vi "Framework_Initialize.vi"(8 "error in (no error)":errorcluster, 11 "AB_Deploy_EXE in":refnum<class "AB_Deploy_EXE.lvclass">) -> (0 "error out":errorcluster, 1 "helpTopics":string[](array[string]), 2 "pageTitles":string[](array[string]), 3 "AB_Deploy_EXE out":refnum<class "AB_Deploy_EXE.lvclass">, 4 "helpFile":string, 5 "pages":path[](array[path]))   [LabVIEW 2020, in "AB_Deploy_EXE.lvclass"]
uses:
  <vilib>/AppBuilder/AB_Classes/DeployableEXE/AB_Deploy_EXE.lvclass
  <vilib>/AppBuilder/AB_Classes/DeployableEXE/AB_Deploy_EXE.lvclass/AB_Deploy_EXE.ctl
  <vilib>/AppBuilder/AB_Classes/EXE/AB_EXE.lvclass
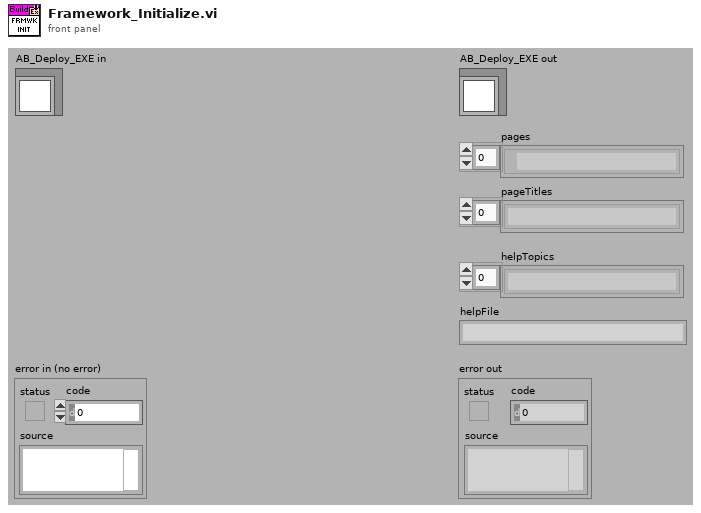
[diagram p1: front panel]
types:
  T1 = enum32{"invalid OS target", "Mac OS", "Windows 3.1", "Windows 95/NT", "Solaris 1", "Solaris 2", "HP-UX", "PowerMAX", "Linux", "Irix", "Rhapsody", "BeOS", "AIX", "OSF1", "VxWorks", "PharLap", "Carbon", "RTX", "Windows x64", "Linux x64", "Mac OS X x64"}
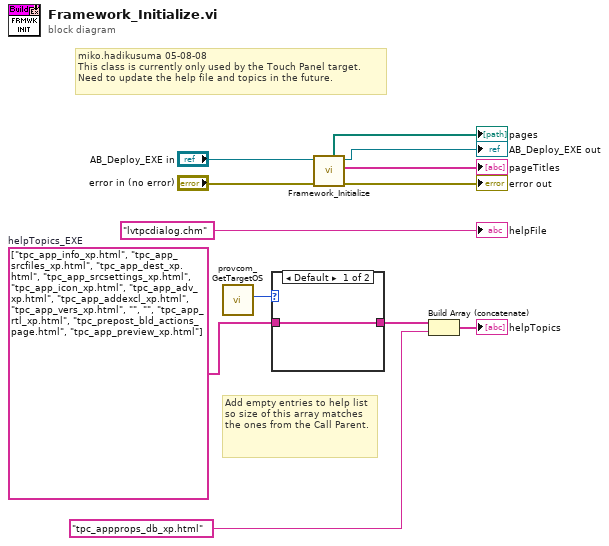
[diagram p0: block diagram]
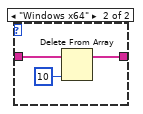
[diagram p2: hidden frame]
diagram:
  w2 = string[] ["tpc_app_info_xp.html", "tpc_app_srcfiles_xp.html", "tpc_app_dest_xp.html", "tpc_app_srcsettings_xp.html", "tpc_app_icon_xp.html", "tpc_app_adv_xp.html", "tpc_app_addexcl_xp.html", "tpc_app_vers_xp.html", "", "", "tpc_app_rtl_xp.html", "tpc_prepost_bld_actions_page.html", "tpc_app_preview_xp.html"]  # helpTopics_EXE
  # "Add empty entries to help list so size of this array matches the ones from the Call Parent."
  # "miko.hadikusuma 05-08-08\nThis class is currently only used by the Touch Panel target.\nNeed to update the help file and topics in the future."
  n1 = call <resource>:"provcom_GetTargetOS.vi"() -> ("App.TargetOS"=w3:T1)  [unwired: 11 out]
  n2 = case shown="Default" w3 {
    tunnel: w2 -> [w13 w16]
    tunnel: [w13 w15] -> w1
    frame Default {
    }
    frame "Windows x64" {
      n3 = Delete From Array(array=w16, index=10) -> (array with subset deleted=w15:string[])  [unwired: 1 in, 1 out]
    }
  }
  n4 = call-parent "Framework_Initialize.vi"("error in (no error)"="error in (no error)", "AB_EXE in"="AB_Deploy_EXE in") -> ("error out"=→"error out":errorcluster, "pageTitles"=→"pageTitles":string[], "AB_EXE out"=→"AB_Deploy_EXE out":refnum<class "AB_Deploy_EXE.lvclass">, "pages"=→"pages":path[])  [unwired: 6 out]
  n5 = Build Array (concatenate)(w1, "tpc_appprops_db_xp.html" ("HTML filename")) -> (→"helpTopics":string[])
  "helpFile" <- "lvtpcdialog.chm" ("CHM or HLP filename (lvdialog.chm)")
